vi "Get NI.LV.Dialog Application Context.vi"(8 "error in (no error)":errorcluster) -> (0 "error out":errorcluster, 3 "Application out":refnum<vi>)   [LabVIEW 2020]
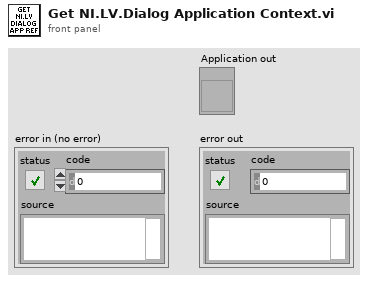
[diagram p1: front panel]
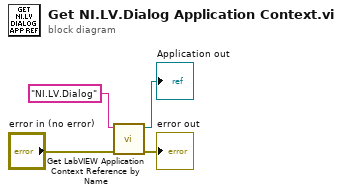
[diagram p0: block diagram]
diagram:
  n1 = call "Get LabVIEW Application Context Reference by Name.vi"("error in (no error)"="error in (no error)", "Context Name"="NI.LV.Dialog") -> ("error out"=→"error out":errorcluster, "Application out"=→"Application out":refnum<vi>)  [unwired: 8 in]
